vi "Queue FGV.vi"(7 "Enum":T1=enum."Get Queue", 8 "error in (no error)":errorcluster) -> (0 "error out":errorcluster, 2 "queue out":refnum<queue>)   [LabVIEW 2013, in "Progress Bar.lvlib"]
uses:
  Progress Bar.lvlib
  Queue Action.ctl
  Property Message.ctl
  Property Action.ctl
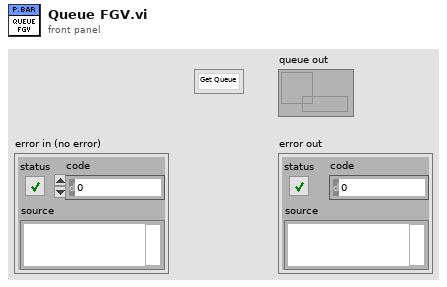
[diagram p1: front panel]
types:
  T1 = typedef "Progress Bar.lvlib/Queue Action.ctl" = enum16{"Obtain Queue", "Release Queue", "Get Queue"}
  T2 = typedef "Progress Bar.lvlib/Property Message.ctl" = cluster{"Property":T3, "Value":variant}
  T3 = typedef "Progress Bar.lvlib/Property Action.ctl" = enum16{"BG Color", "Title Text Color", "Title Text", "Action Text Color", "Action Text", "Bar Color", "Set Slider Value", "Add to Slider Value", "Exit"}
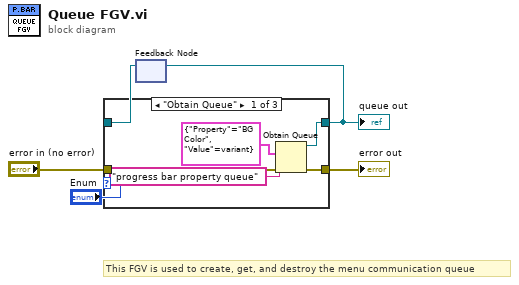
[diagram p0: block diagram]
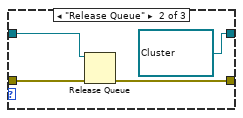
[diagram p2: hidden frame]
diagram:
  # "This FGV is used to create, get, and destroy the menu communication queue"
  n1 = feedback #1() -> (w3:refnum<queue>)  [unwired: 1 in]
  n2 = case shown="\"Obtain Queue\"" "Enum" {
    tunnel: [w9 refnum<queue> refnum ("queue out") w16] -> w4
    tunnel: w3 -> [_ w14 w16]
    tunnel: [w7 w12 w15] -> w2
    tunnel: "error in (no error)" -> [w8 w11 w15]
    frame "Obtain Queue" {
      n3 = Obtain Queue(name (unnamed)="progress bar property queue", element data type=T2 {"Property"=enum."BG Color", "Value"=variant} ("Cluster"), error in (no error)=w8) -> (queue out=w9:refnum<queue>, error out=w7:errorcluster)  [unwired: 2 in, 1 out]
    }
    frame "Release Queue" {
      n4 = Release Queue(queue=w14, error in (no error)=w11) -> (error out=w12:errorcluster)  [unwired: 1 in, 2 out]
    }
    frame "Get Queue" {
    }
  }
  "queue out" <- w4
  "error out" <- w2
  n5 = feedback-in #1(w4) -> ()
